vi "UE9 eDO Example.vi"() -> (0 "error out":errorcluster)   [LabVIEW 2021]
panel:
  in  "Address":string="192.168.1.209"
  in  "ConnectionType":u16(ring) items=["LJ_ctUSB", "LJ_ctETHERNET"]
  in  "FirstFound":bool=TRUE
  in  "State":bool
  in  "Channel":i32
  out "Error Message":string
  # "Sets 1 digital output using the UD easy function eDO."
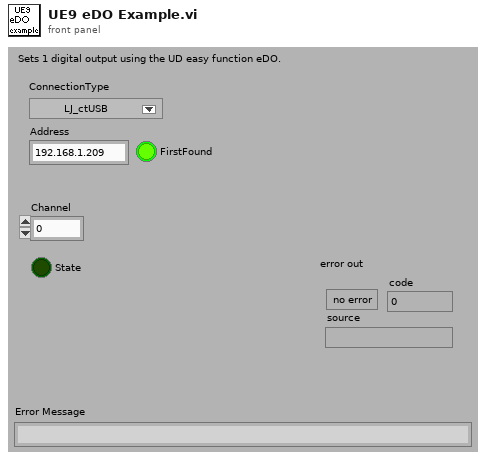
[diagram p1: front panel]
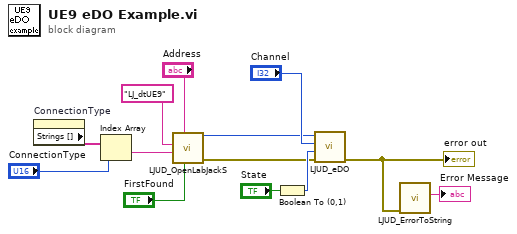
[diagram p0: block diagram]
diagram:
  n1 = property on="ConnectionType" class="Ring (strict)"() -> ("Strings []"=w8:string[])  [unwired: 2 in, 2 out]
  n2 = Index Array(array=w8, index="ConnectionType") -> (element=w4:string)
  n3 = call "LJUD_OpenLabJackS.vi"("FirstFound"="FirstFound", "Address"="Address", "ConnectionType"=w4, "DeviceType"="LJ_dtUE9") -> ("error out"=w1:errorcluster, "Handle"=w2:i32)  [unwired: 5 in, 1 out]
  n4 = Boolean To (0,1)(Boolean="State") -> (0, 1=w9:i16)
  n5 = call "LJUD_eDO.vi"("error in"=w1, "State"=w9, "Channel"="Channel", "Handle In"=w2) -> ("error out"=w12:errorcluster)  [unwired: 6 in, 1 out]
  "error out" <- w12
  n6 = call "LJUD_ErrorToString.vi"("error in"=w12) -> ("String"=→"Error Message":string)  [unwired: 10 in]
